vi "Pockels Cal-Window size and picture.vi"(8 "error in (no error)":errorcluster, 9 "Original window size":cluster{"Horisontal":i16, "Vertical":i16}, 11 "State":T1) -> (0 "error out":errorcluster)   [LabVIEW 2020]
uses:
  Typedefs/Pockels cal wizard states.ctl
  Typedefs/Colapsed-Expanded.ctl
  Globals/gl_Calibration globals.vi
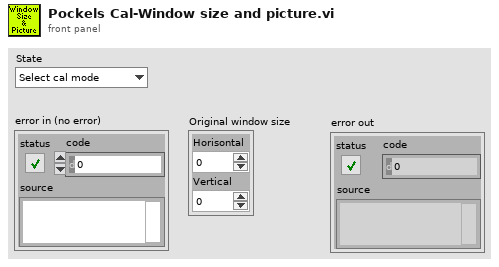
[diagram p1: front panel]
types:
  T1 = typedef "Pockels cal wizard states.ctl" = enum16{"Select cal mode", "Show instructions 1", "Select channel", "Show instructions 2", "Show instructions 3", "Confirm start", "Start calibration"}
  T2 = typedef "Pre-AOL Z wizard refs.ctl" = cluster{"VI's reference":refnum<vi>, "Calibration Mode":refnum<vi>, "Cal points":refnum<vi>, "Channel Selector":refnum<vi>, "Message":refnum<vi>, "Back":refnum<vi>, "Next":refnum<vi>, "Power meter AI":refnum<vi>, "2D Picture":refnum<vi>, "Note":refnum<vi>}
  T3 = typedef "Colapsed-Expanded.ctl" = enum16{"Original size", "Expanded-Size A"}
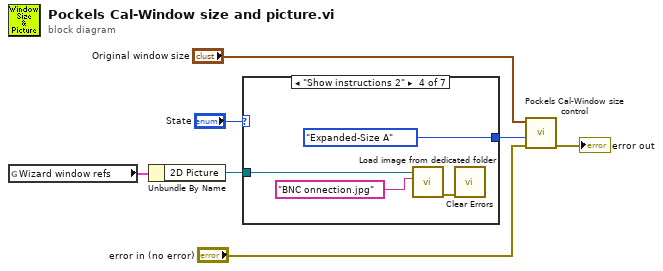
[diagram p0: block diagram]
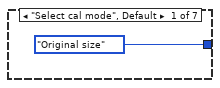
[diagram p2: hidden frame]
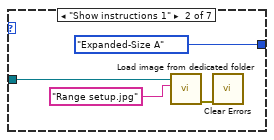
[diagram p3: hidden frame]
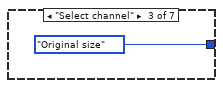
[diagram p4: hidden frame]
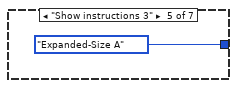
[diagram p5: hidden frame]
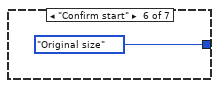
[diagram p6: hidden frame]
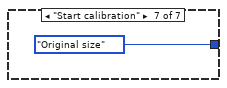
[diagram p7: hidden frame]
diagram:
  n1 = global read "gl_Calibration globals.vi" "Wizard window refs"() -> (w2:T2)
  n2 = Unbundle By Name(w2) -> ("2D Picture"=w1:refnum<vi>)
  n3 = case shown="\"Show instructions 2\"" "State" {
    tunnel: [Colapsed-Expanded."Original size" ("Function") Colapsed-Expanded."Expanded-Size A" ("Function") Colapsed-Expanded."Original size" ("Function") Colapsed-Expanded."Expanded-Size A" ("Function") Colapsed-Expanded."Expanded-Size A" ("Function") Colapsed-Expanded."Original size" ("Function") Colapsed-Expanded."Original size" ("Function")] -> w6
    tunnel: w1 -> [_ w11 _ w14 _ _ _]
    frame "Select cal mode", Default {
    }
    frame "Show instructions 1" {
      n4 = call "Load image from dedicated folder.vi"("name or relative path"="Range setup.jpg", "2D Picture ctrl ref"=w11) -> ("error out"=w9:errorcluster)  [unwired: 9 in]
      n5 = call <vilib>:"Clear Errors.vi"("error in (no error)"=w9) -> ()  [unwired: 5 in, 2 out]
    }
    frame "Select channel" {
    }
    frame "Show instructions 2" {
      n6 = call "Load image from dedicated folder.vi"("name or relative path"="BNC onnection.jpg", "2D Picture ctrl ref"=w14) -> ("error out"=w15:errorcluster)  [unwired: 9 in]
      n7 = call <vilib>:"Clear Errors.vi"("error in (no error)"=w15) -> ()  [unwired: 5 in, 2 out]
    }
    frame "Show instructions 3" {
    }
    frame "Confirm start" {
    }
    frame "Start calibration" {
    }
  }
  n8 = call "Pockels Cal-Window size control.vi"("error in (no error)"="error in (no error)", "Function"=w6, "Original window size"="Original window size") -> ("error out"=→"error out":errorcluster)  [unwired: 8 in]
